vi "Buffer Capacity.vi"(8 "error in (no error)":errorcluster, 9 "Buffer Name":string, 11 "VISA resource name":refnum<visa-resource-name>) -> (0 "error out":errorcluster, 1 "Capacity":u32, 3 "VISA resource name out":refnum<visa-resource-name>, 4 "Command String":string)   [LabVIEW 2009, in "Keithley 2600 Series.lvlib"]
doc: "This VI queries the capacity of the reading buffer.\n\n<b>Functions and Attributes Used</b>\n<buffername>.capacity"
uses:
  <instrlib>/Keithley 2600 Series/Keithley 2600 Series.lvlib
  <instrlib>/Keithley 2600 Series/Private/GlobalVariables.vi
panel:
  # "(c) 2008 Keithley Instruments, Inc.  ALL RIGHTS RESERVED."
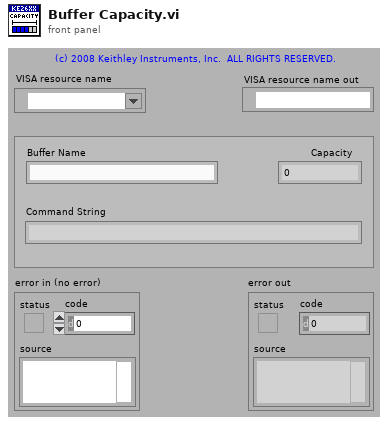
[diagram p1: front panel]
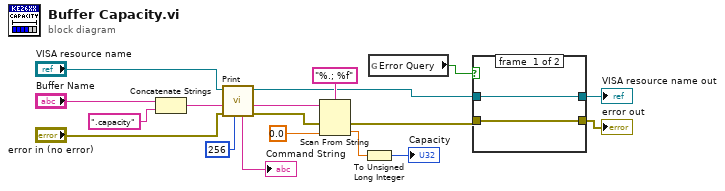
[diagram p0: block diagram]
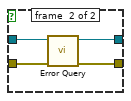
[diagram p2: hidden frame]
diagram:
  n1 = Concatenate Strings("Buffer Name", ".capacity" ("command")) -> (w8:string)
  n2 = call <instrlib>:"Print.vi"("Byte Count (1024)"=u32 256, "error in (no error)"="error in (no error)", "Input"=w8, "VISA resource name"="VISA resource name") -> ("error out"=w3:errorcluster, "Output"=w4:string, "VISA resource name out"=w2:refnum<visa-resource-name>, "Command String"=→"Command String":string)  [unwired: 1 in, 3 out]
  n3 = Scan From String(format string="%.; %f", input string=w4, error in=w3, default 1=0.0 ("default value 1")) -> (error out=w12:errorcluster, output 1=w15:dbl)  [unwired: 1 in, 2 out]
  n4 = To Unsigned Long Integer(number=w15) -> (unsigned 32bit integer=→"Capacity":u32)
  n5 = global read "GlobalVariables.vi" "Error Query"() -> (w13:bool)
  n6 = case shown="True" w13 {
    tunnel: w12 -> [w20 w24]
    tunnel: [w19 w23] -> w11
    tunnel: [w20 w22] -> w10
    tunnel: w2 -> [w19 w21]
    frame #0 {
    }
    frame #1 {
      n7 = call <instrlib>:"Error Query.vi"("error in (no error)"=w24, "VISA resource name"=w21) -> ("error out"=w22:errorcluster, "VISA resource name out"=w23:refnum<visa-resource-name>)  [unwired: 8 out]
    }
  }
  "VISA resource name out" <- w11
  "error out" <- w10
